vi "Test Boolean.vi"() -> (0 "error out":errorcluster, 3 "Pass":bool)   [LabVIEW 2021]
uses:
  Boolean_CIF_U.lvlib
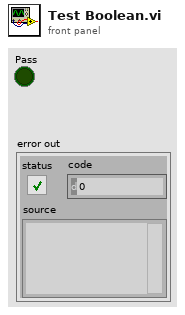
[diagram p1: front panel]
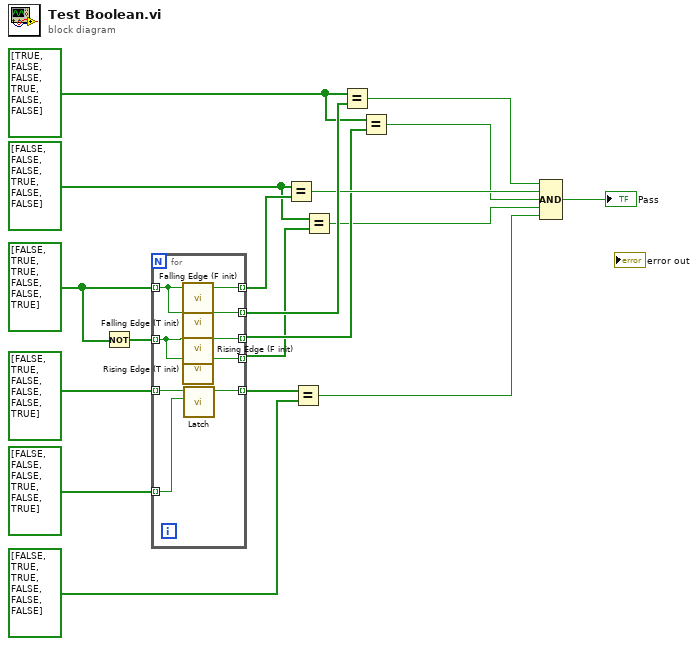
[diagram p0: block diagram]
diagram:
  w11 = bool[] [TRUE, FALSE, FALSE, TRUE, FALSE, FALSE] ("Array 2")
  w9 = bool[] [FALSE, FALSE, FALSE, TRUE, FALSE, FALSE] ("Array 2")
  w13 = bool[] [FALSE, TRUE, TRUE, FALSE, FALSE, TRUE]
  n1 = Not(x=w13) -> (.not. x?=w12:bool[])
  n2 = for {
    tunnel: w13 -> [w26] mode=indexing
    tunnel: [w27] -> w18 mode=indexing
    tunnel: [w25] -> w17 mode=indexing
    tunnel: w12 -> [w24] mode=indexing
    tunnel: [w23] -> w10 mode=indexing
    tunnel: [w22] -> w8 mode=indexing
    tunnel: bool[] [FALSE, TRUE, FALSE, FALSE, FALSE, TRUE] -> [w21] mode=indexing
    tunnel: bool[] [FALSE, FALSE, FALSE, TRUE, FALSE, TRUE] -> [w20] mode=indexing
    tunnel: [w19] -> w3 mode=indexing
    n3 = call "Falling Edge (F init).vi"("Signal"=w26) -> ("Edge Detected"=w27:bool)  [unwired: 4 in]
    n4 = call "Falling Edge (T init).vi"("Signal"=w26) -> ("Edge Detected"=w25:bool)  [unwired: 4 in]
    n5 = call "Rising Edge (F init).vi"("Signal"=w24) -> ("Edge Detected"=w23:bool)  [unwired: 4 in]
    n6 = call "Rising Edge (T init).vi"("Signal"=w24) -> ("Edge Detected"=w22:bool)  [unwired: 4 in]
    n7 = call "Latch.vi"("clear"=w20, "set"=w21) -> ("out"=w19:bool)  [unwired: 9 in]
  }
  n8 = Equal?(x=w9, y=w18) -> (x = y?=w14:bool)
  n9 = Equal?(x=w3, y=bool[] [FALSE, TRUE, TRUE, FALSE, FALSE, FALSE] ("Array 2")) -> (x = y?=w1:bool)
  n10 = Equal?(x=w9, y=w8) -> (x = y?=w7:bool)
  n11 = Equal?(x=w11, y=w17) -> (x = y?=w15:bool)
  n12 = Equal?(x=w11, y=w10) -> (x = y?=w6:bool)
  n13 = Compound Arithmetic op=AND(w15, w14, w6, w7, w1) -> (→"Pass":bool)
